vi "MuxCardSwitch.vi"(6 "Single Needle":bool, 7 "Probe Card Channels":i32=32, 8 "error in (no error)":errorcluster, 9 "disabled channels":u32[](array[numeric]), 10 "Switch to channel":i32, 11 "Pickering in":refnum<class "Pickering.lvclass">) -> (0 "error out":errorcluster, 2 "last channel no.":i32, 3 "Pickering out":refnum<class "Pickering.lvclass">)   [LabVIEW 2013, in "Pickering.lvclass"]
uses:
  Pickering.lvclass
  InstrumentSetup.vi
  InstrControl.lvclass
panel:
  out "Display Matrix":bool[][](array[boolean])
  # "Pickering Multiplexer Settings"
  # "X1"
  # "X2"
  # "X3"
  # "X4"
  # "X5"
  # "X6"
  # "X7"
  # "X8"
  # "Y1  Y2  Y3  Y4"
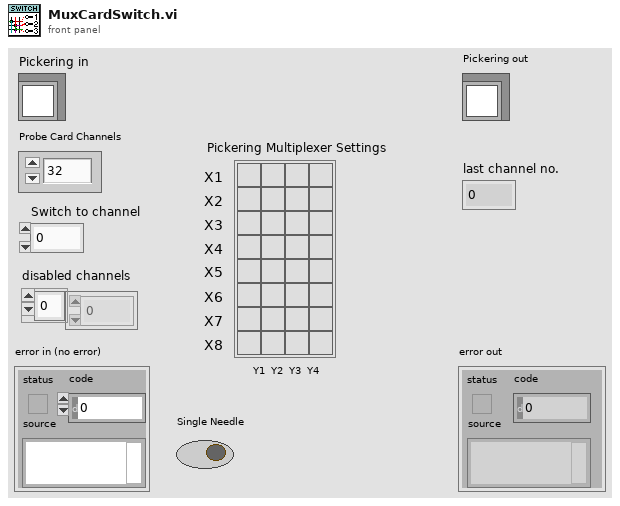
[diagram p1: front panel]
types:
  T1 = cluster{"Matrix address":string, "Mux1 address":string, "Mux2 address":string, "Matrix used?":bool, "Switching":refnum<class "Pickering.lvclass">, "Matrix X Channels":cluster{"Bias Supply / SMU LO":i32, "Bias Supply / SMU HI":i32, "CV Box LO":i32, "CV Box HI":i32, "CV Box LO IN":i32, "CV Box HI IN":i32, "Volt meter LO":i32, "Volt meter HI":i32, "Mux1 C1":i32, "Mux1 C2":i32, "Mux2 C1":i32, "Mux2 C2":i32}}
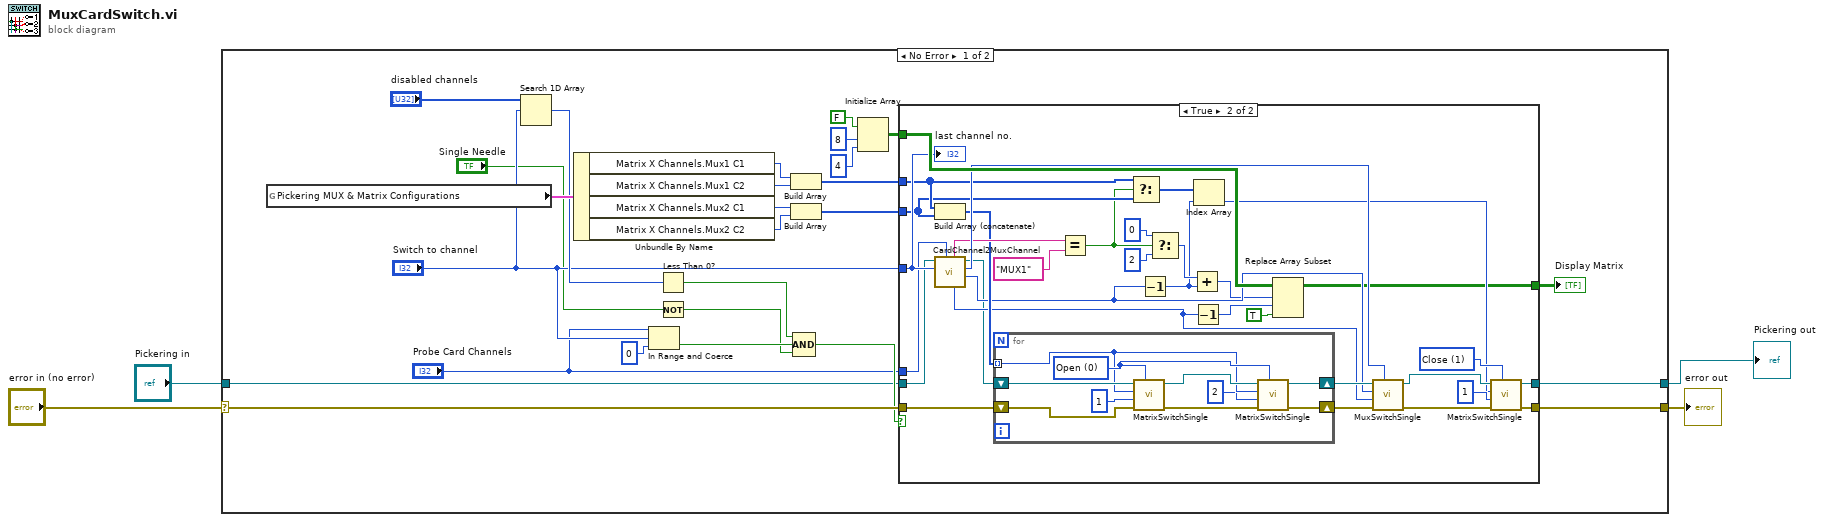
[diagram p0: block diagram]
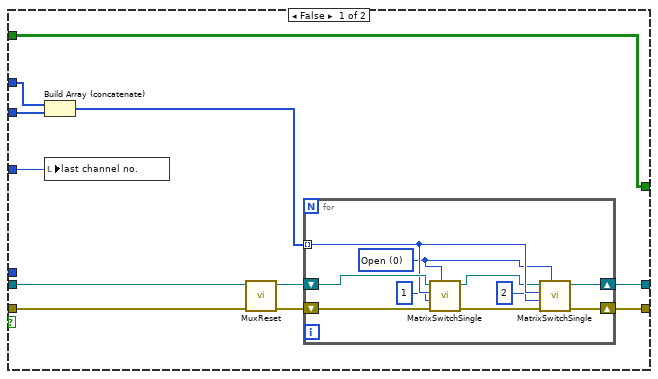
[diagram p2: hidden frame]
diagram:
  n1 = case shown="No Error" "error in (no error)" {
    selector: "error in (no error)" -> [w29 w96]
    tunnel: [w24 w96] -> w3
    tunnel: [w8 w95] -> w2
    tunnel: "Pickering in" -> [w7 w95]
    frame No Error {
      n2 = global read "InstrumentSetup.vi" "Pickering MUX & Matrix Configurations"() -> (w30:T1)
      n3 = Search 1D Array(1D array="disabled channels", element="Switch to channel") -> (index of element=w21:i32)  [unwired: 1 in]
      n4 = Unbundle By Name(w30) -> ("Matrix X Channels.Mux1 C1"=w26:i32, "Matrix X Channels.Mux1 C2"=w25:i32, "Matrix X Channels.Mux2 C1"=w27:i32, "Matrix X Channels.Mux2 C2"=w28:i32)
      n5 = In Range and Coerce(upper limit="Probe Card Channels", x="Switch to channel", lower limit=0) -> (In Range?=w19:bool)  [unwired: 1 out]
      n6 = Less Than 0?(x=w21) -> (x < 0?=w20:bool)
      n7 = Not(x="Single Needle") -> (.not. x?=w18:bool)
      n8 = Build Array(w26, w25) -> (w11:i32[])
      n9 = Build Array(w27, w28) -> (w10:i32[])
      n10 = Compound Arithmetic op=AND(w20, w19, w18) -> (w17:bool)
      n11 = Initialize Array(FALSE, 8, 4) -> (w12:bool[][])
      n12 = case shown="True" w17 {
        tunnel: "Switch to channel" -> [w41 w76]
        tunnel: w7 -> [w40 w54]
        tunnel: w29 -> [w37 w84]
        tunnel: [w36 w65] -> w24
        tunnel: w12 -> [w32 w77]
        tunnel: w11 -> [w35 w70]
        tunnel: w10 -> [w34 w69]
        tunnel: [w32 w56] -> w9
        tunnel: [w31 w55] -> w8
        tunnel: "Probe Card Channels" -> [_ w52]
        frame False {
          n13 = Build Array (concatenate)(w35, w34) -> (w33:i32[])
          n14 = local write "last channel no."(w41) -> ()
          n15 = call-dynamic "MuxReset.vi"("error in (no error)"=w37, "Pickering in"=w40) -> ("error out"=w38:errorcluster, "Pickering out"=w39:refnum<class "Pickering.lvclass">)  [unwired: 8 in]
          n16 = for {
            tunnel: w33 -> [w49] mode=indexing
            shift-right: [w48] -> w36
            shift-left: w38 -> [w50]
            shift-right: [w42] -> w31
            shift-left: w39 -> [w51]
            w47 = u16 0 items=["Open", "Close"] ("Switch action")
            n17 = call-dynamic "MatrixSwitchSingle.vi"("Switch action"=w47, "error in (no error)"=w50, "Matrix Y"=1, "Matrix X"=w49, "Pickering in"=w51) -> ("error out"=w45:errorcluster, "Pickering out"=w46:refnum<class "Pickering.lvclass">)  [unwired: 4 in, 1 out]
            n18 = call-dynamic "MatrixSwitchSingle.vi"("Switch action"=w47, "error in (no error)"=w45, "Matrix Y"=2, "Matrix X"=w49, "Pickering in"=w46) -> ("error out"=w48:errorcluster, "Pickering out"=w42:refnum<class "Pickering.lvclass">)  [unwired: 4 in, 1 out]
          }
        }
        frame True {
          w81 = u16 1 items=["Open", "Close"] ("Switch action")
          n19 = Build Array (concatenate)(w70, w69) -> (w68:i32[])
          n20 = call-dynamic "CardChannel2MuxChannel.vi"("Probe Card Channels"=w52, "Probecard Channel No."=w76, "Pickering in"=w54) -> ("C1 / C2"=w59:i32, "Mux No.:"=w73:u32, "Pickering out"=w53:refnum<class "Pickering.lvclass">, "Channel"=w64:i32, "Mux No. string"=w71:string)  [unwired: 3 in, 1 out]
          n21 = for {
            tunnel: w68 -> [w88] mode=indexing
            shift-right: [w92] -> w75
            shift-left: w84 -> [w94]
            shift-right: [w85] -> w74
            shift-left: w53 -> [w91]
            w89 = u16 0 items=["Open", "Close"] ("Switch action")
            n22 = call-dynamic "MatrixSwitchSingle.vi"("Switch action"=w89, "error in (no error)"=w94, "Matrix Y"=1, "Matrix X"=w88, "Pickering in"=w91) -> ("error out"=w93:errorcluster, "Pickering out"=w90:refnum<class "Pickering.lvclass">)  [unwired: 4 in, 1 out]
            n23 = call-dynamic "MatrixSwitchSingle.vi"("Switch action"=w89, "error in (no error)"=w93, "Matrix Y"=2, "Matrix X"=w88, "Pickering in"=w90) -> ("error out"=w92:errorcluster, "Pickering out"=w85:refnum<class "Pickering.lvclass">)  [unwired: 4 in, 1 out]
          }
          n24 = Equal?(x=w71, y="MUX1") -> (x = y?=w63:bool)
          n25 = Select(t=w70, s=w63, f=w69) -> (s? t:f=w67:i32[])
          n26 = Decrement(x=w59) -> (x-1=w57:i32)
          n27 = Select(t=0, s=w63, f=2) -> (s? t:f=w60:i32)
          n28 = Add(x=w60, y=w57) -> (x+y=w58:i32)
          n29 = Decrement(x=w64) -> (x-1=w79:i32)
          n30 = Index Array(array=w67, index=w57) -> (element=w66:i32)
          n31 = Replace Array Subset(array=w77, new element=TRUE, index (row)=w58, index (col)=w79) -> (w56:bool[][])
          n32 = call-dynamic "MuxSwitchSingle.vi"("MUX address"=w73, "error in (no error)"=w75, "Channel"=w64, "C1 / C2"=w59, "Pickering in"=w74) -> ("error out"=w83:errorcluster, "Pickering out"=w82:refnum<class "Pickering.lvclass">)  [unwired: 4 in, 1 out]
          n33 = call-dynamic "MatrixSwitchSingle.vi"("Switch action"=w81, "error in (no error)"=w83, "Matrix Y"=1, "Matrix X"=w66, "Pickering in"=w82) -> ("error out"=w65:errorcluster, "Pickering out"=w55:refnum<class "Pickering.lvclass">)  [unwired: 4 in, 1 out]
          "last channel no." <- w76
        }
      }
      "Display Matrix" <- w9
    }
    frame Error {
    }
  }
  "error out" <- w3
  "Pickering out" <- w2
